vi "计算三角形内心与半径.vi"(8 "Error In":errorcluster caption="错误输入", 11 "三角形":T1) -> (0 "Error Out":errorcluster caption="错误输出", 2 "半径":dbl, 3 "内心":T2)   [LabVIEW 2012, in "几何工具.lvlib"]
uses:
  <vilib>/Utility/miscctls.llb/LVPointDoubleTypeDef.ctl
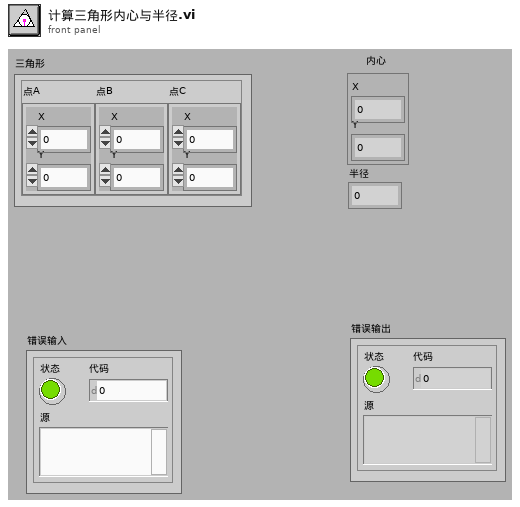
[diagram p1: front panel]
types:
  T1 = typedef "几何工具.lvlib/三角形.ctl" = cluster{"点A":T2, "点B":T2, "点C":T2}
  T2 = typedef "LVPointDoubleTypeDef.ctl" = cluster{"X":dbl, "Y":dbl}
  T3 = typedef "几何工具.lvlib/斜率与截距.ctl" = cluster{"斜率":dbl, "截距":dbl}
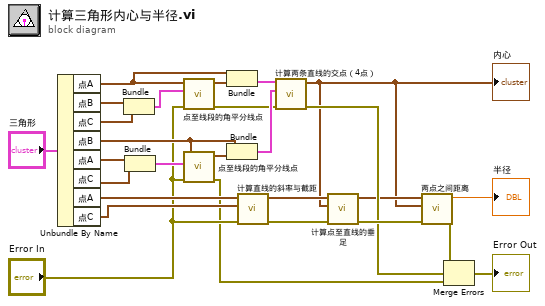
[diagram p0: block diagram]
diagram:
  n1 = Unbundle By Name("三角形") -> ("点A"=w23:T2, "点B"=w26:T2, "点C"=w25:T2, "点B"=w17:T2, "点A"=w20:T2, "点C"=w19:T2, "点A"=w15:T2, "点C"=w14:T2)
  n2 = Bundle("点B"=w26, "点C"=w25) -> (w24:cluster{"点B":T2, "点C":T2})  [unwired: 1 in]
  n3 = Bundle("点A"=w20, "点C"=w19) -> (w18:cluster{"点A":T2, "点C":T2})  [unwired: 1 in]
  n4 = call "点至线段的角平分线点.vi"("Error In"="Error In", "线段"=w24, "点A"=w23) -> ("Error Out"=w7:errorcluster, "角平分线点"=w22:T2)  [unwired: 7 in]
  n5 = call "点至线段的角平分线点.vi"("Error In"="Error In", "线段"=w18, "点A"=w17) -> ("Error Out"=w6:errorcluster, "角平分线点"=w16:T2)  [unwired: 7 in]
  n6 = Bundle("点A"=w23, "角平分线点"=w22) -> (w21:cluster{"点A":T2, "角平分线点":T2})  [unwired: 1 in]
  n7 = Bundle("点B"=w17, "角平分线点"=w16) -> (w11:cluster{"点B":T2, "角平分线点":T2})  [unwired: 1 in]
  n8 = call "计算直线的斜率与截距.vi"("Error In"="Error In", "点B"=w14, "点A"=w15) -> ("Error Out"=w9:errorcluster, "斜率与截距"=w13:T3)  [unwired: 7 in]
  n9 = call "计算两条直线的交点（4点）.vi"("Error In"=w7, "直线B"=w11, "直线A"=w21) -> ("Error Out"=w5:errorcluster, "交点"=w1:T2)  [unwired: 7 in]
  "内心" <- w1
  n10 = call "计算点至直线的垂足.vi"("Error In"=w9, "Point"=w1, "直线"=w13) -> ("Error Out"=w8:errorcluster, "垂足点"=w2:T2)  [unwired: 7 in]
  n11 = call "两点之间距离.vi"("Error In"=w8, "点B"=w1, "点A"=w2) -> ("Error Out"=w3:errorcluster, "距离AB"=→"半径":dbl)  [unwired: 7 in]
  n12 = Merge Errors(w3, w5, w6) -> (→"Error Out":errorcluster)
